vi "Autonomous.vi"() -> ()   [LabVIEW 2020]
doc: "This VI starts when autonomous period begins, and will automatically be terminated when it ends. You can carry out timed or sensor driven operations directly to I/O or to subsystems without needing to return to the caller."
uses:
  <vilib>/Rock Robotics/WPI/Framework/Command Status Info.ctl
  <vilib>/Rock Robotics/WPI/Framework/Completion Status.ctl
  <vilib>/Rock Robotics/WPI/Framework/Completion Notifier.ctl
  Swerve/Implementation/Swerve Operations.ctl
  Swerve/Implementation/Swerve Setpoints.ctl
  <vilib>/Rock Robotics/WPI/Utilities/WPI_GetSetVariantRefNum.vi
  <vilib>/Rock Robotics/Network Tables/NT Read String.vi
panel:
  out "Command Info Out 3":T1
  out "Command Info Out 2":T1
  out "Command Info Out":T1
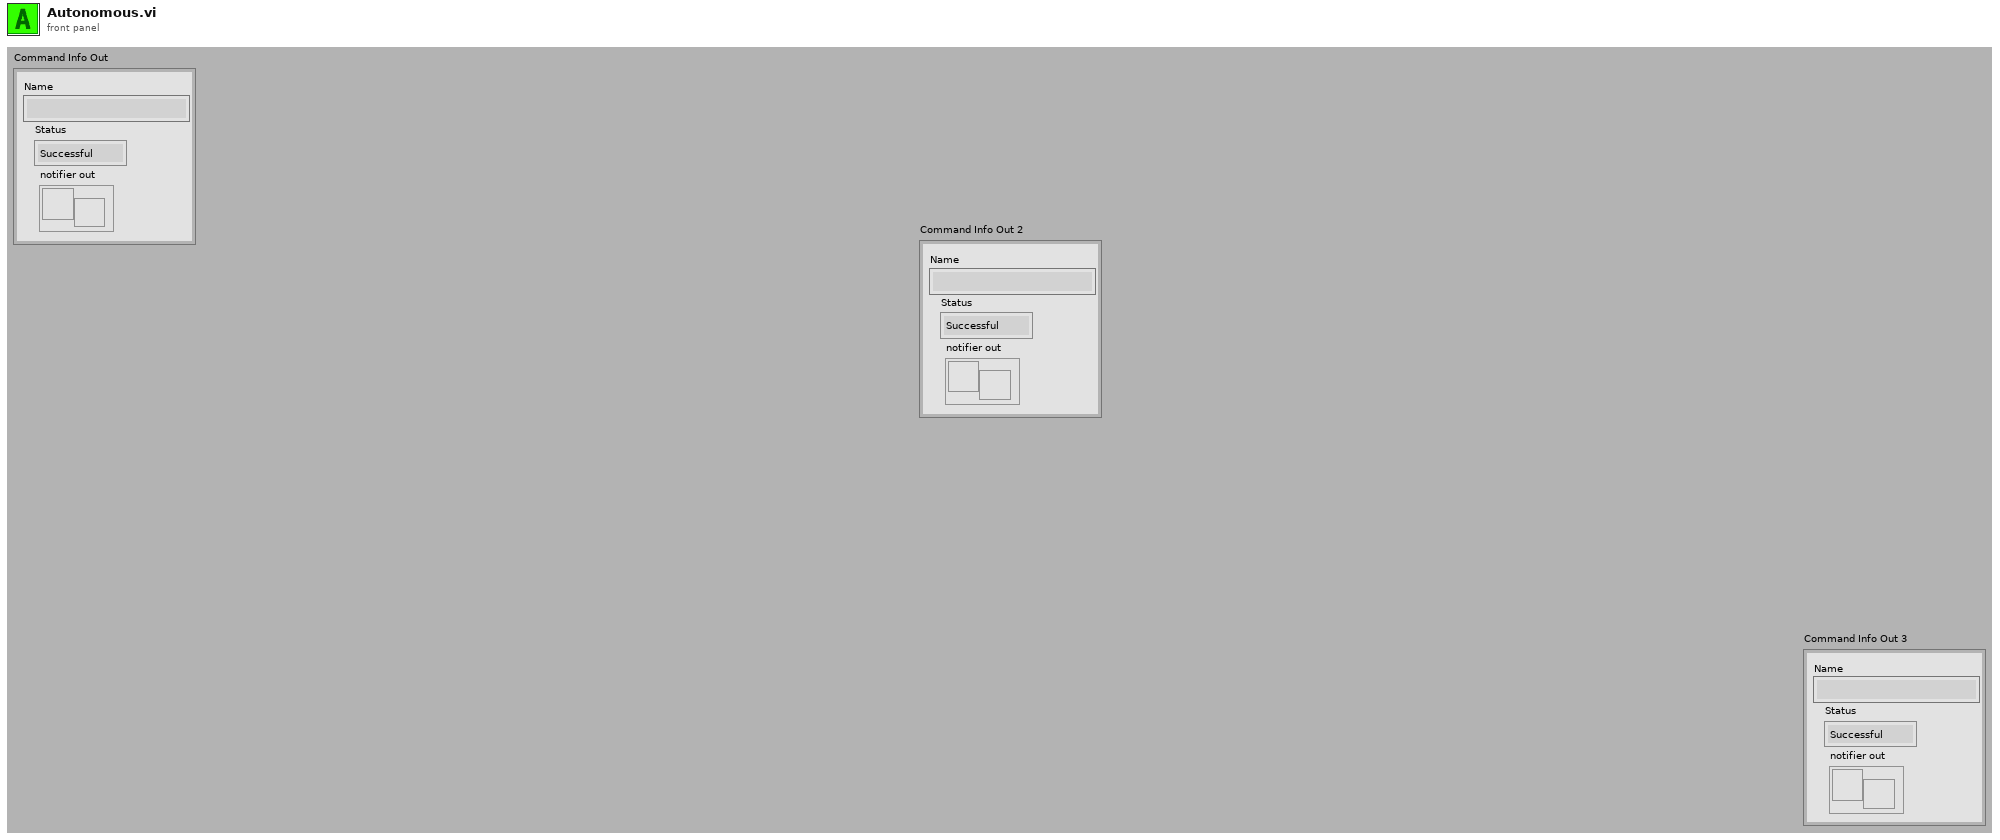
[diagram p1: front panel]
types:
  T1 = typedef "Command Status Info.ctl" = cluster{"Name":string, "Status":T2, "notifier out":T3}
  T2 = typedef "Completion Status.ctl" = enum16{"Successful", "Aborted", "Incomplete"}
  T3 = typedef "Completion Notifier.ctl" = refnum<notifier>
  T4 = typedef "WPI_JoystickDevRef.ctl" = cluster{"Device":T5}
  T5 = typedef "WPI_JoystickDeviceEnum.ctl" = enum16{"USB 0", "USB 1", "USB 2", "USB 3", "USB 4", "USB 5"}
  T6 = typedef "Swerve Setpoints.ctl" = cluster{"Operation":T7, "Gyro":dbl, "X Rotate":dbl, "FWD":dbl, "STR":dbl, "Time":dbl, "Angle":dbl, "Distance":dbl, "Right Trigger":dbl, "Y Rotate":dbl, "Start Angle":dbl}
  T7 = typedef "Swerve Operations.ctl" = enum16{"Reserve", "Read Current", "Immediate", "Direct  Joystick Drive", "Joystick Drive", "Drive for Distance", "Drive for Time", "Turn to Angle", "Drive to Angle(Time)", "Drive to Angle(Distance)"}
  T8 = typedef "WPI_MotorControlDeviceRef.ctl" = cluster{"DeviceStatus":errorcluster, "Type":T9, "PWM":cluster{"PWM Channel":T10, "DeadBand":T11}, "CAN":cluster{"Device Number":u8, "SetOutput VI Ref":variant, "GetOutput VI Ref":variant, "Enable VI Ref":variant, "Disable VI Ref":variant, "Data":variant}, "Invert":bool, "DIO PWM":cluster{"PWM \"Enable\" Channel":T10, "DIOChannel":T12, "PWM Rate":dbl}}
  T9 = typedef "WPI_MotorControlType.ctl" = enum16{"PWM", "CAN", "DIO PWM"}
  T10 = typedef "FPGA_DIOPWMChannel.ctl" = enum8{"PWM 0", "PWM 1", "PWM 2", "PWM 3", "PWM 4", "PWM 5", "PWM 6", "PWM 7", "PWM 8", "PWM 9", "PWM MXP 0", "PWM MXP 1", "PWM MXP 2", "PWM MXP 3", "PWM MXP 4", "PWM MXP 5", "PWM MXP 6", "PWM MXP 7", "PWM MXP 8", "PWM MXP 9", "Invalid"}
  T11 = typedef "WPI_PWMDeadband.ctl" = cluster{"Name":string, "maxPositivePwm":i32, "minPositivePwm":i32, "centerPwm":i32, "maxNegativePwm":i32, "minNegativePwm":i32, "angularRange":u16}
  T12 = typedef "FPGA_DIOChannel.ctl" = enum8{"DIO 0", "DIO 1", "DIO 2", "DIO 3", "DIO 4", "DIO 5", "DIO 6", "DIO 7", "DIO 8", "DIO 9", "DIO MXP 0", "DIO MXP 1", "DIO MXP 2", "DIO MXP 3", "DIO MXP 4", "DIO MXP 5", "DIO MXP 6", "DIO MXP 7", "DIO MXP 8", "DIO MXP 9", "DIO MXP 10", "DIO MXP 11", "DIO MXP 12", "DIO MXP 13", "DIO MXP 14", "DIO MXP 15", "SPI Port CS1", "SPI Port CS2", "SPI Port CS3", "SPI Port MISO", "SPI Port MOSI", "Invalid"}
  T13 = typedef "ADIS16470 Device Reference.ctl" = cluster{"DevStatus":errorcluster, "Hardware Config":T14, "Calibration Complete":refnum<notifier>, "Status Reference":refnum<data-value>, "Data Reference":refnum<data-value>, "Sychronous Process VI":T17, "Cmd FIFO":refnum<k33>, "Source":T18, "Data FIFO":refnum<k33>, "Calibration Time (ms)":u32, "Data Reference":refnum<data-value>}
  T14 = typedef "ADIS16470 Hardware Configuration.ctl" = cluster{"SPI Clock Rate (Hz)":dbl, "IMU SPI Mode (3)":T15, "IMU Reset Pin":T12, "IMU SPI Bus":T16, "IMU Data Ready Pin":T12, "Stall Config":cluster{"Pow2BytesPerRead":u8, "StallTicks":u16, "CsToSclkTicks":u8}}
  T15 = typedef "WPI_SPIMode.ctl" = enum16{"Mode 0 (Clk Idle Low,Sample on Leading)", "Mode 1 (Clk Idle Low,Sample on Trailing)", "Mode 2 (Clk Idle High,Sample on Leading)", "Mode 3 (Clk Idle High,Sample on Trailing)"}
  T16 = typedef "spi_bus.ctl" = enum16{"SPI On-Board, CS0", "SPI On-Board, CS1", "SPI On-Board, CS2", "SPI On-Board, CS3", "SPI MXP", "Invalid"}
  T17 = typedef "ADIS16470 Process.ctl" = refnum<vi>
  T18 = typedef "FPGA_CounterEncoderSourceConvertionLVSourceType.ctl" = cluster{"DevStatus":errorcluster, "AnalogTriggerMode?":bool, "DigitalMode":cluster{"DIO Channel":T19}, "AnalogTriggerMode":cluster{"AnalogTriggerIndex":T20, "OutputType":T21}}
  T19 = typedef "FPGA_DIODigitalSourceChannel.ctl" = enum8{"DIO 0", "DIO 1", "DIO 2", "DIO 3", "DIO 4", "DIO 5", "DIO 6", "DIO 7", "DIO 8", "DIO 9", "DIO MXP 0", "DIO MXP 1", "DIO MXP 2", "DIO MXP 3", "DIO MXP 4", "DIO MXP 5", "DIO MXP 6", "DIO MXP 7", "DIO MXP 8", "DIO MXP 9", "DIO MXP 10", "DIO MXP 11", "DIO MXP 12", "DIO MXP 13", "DIO MXP 14", "DIO MXP 15", "SPI Port CS1", "SPI Port CS2", "SPI Port CS3", "SPI Port MISO", "SPI Port MOSI", "Disabled"}
  T20 = typedef "FPGA_AnalogTriggerIndex.ctl" = enum8{"Trig 0", "Trig 1", "Trig 2", "Trig 3", "Trig 4", "Trig 5", "Trig 6", "Trig 7", "Invalid"}
  T21 = typedef "FPGA_AnalogTriggerOutType.ctl" = enum16{"InWindow", "TriggerState", "Rising", "Falling"}
  T22 = typedef "ADIS16470 Data.ctl" = cluster{"XAngle":dbl, "YAngle":dbl, "ZAngle":dbl}
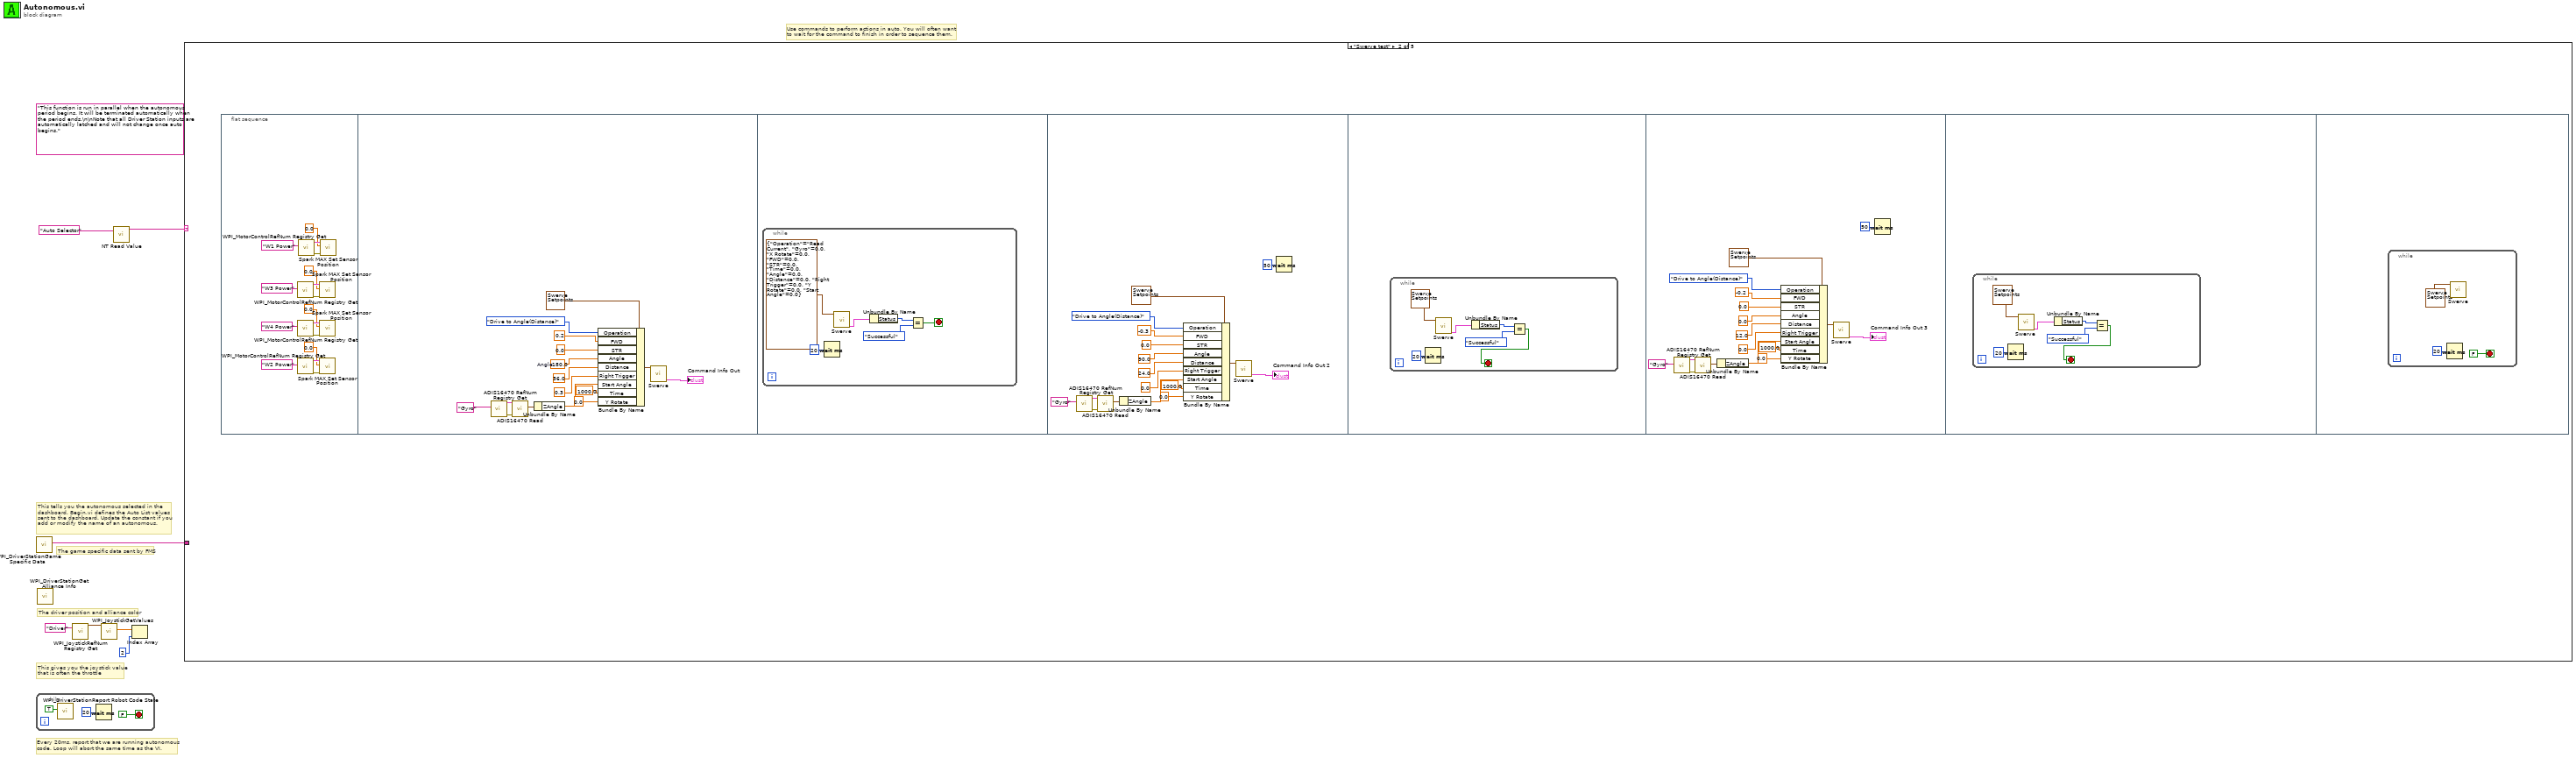
[diagram p0: block diagram]
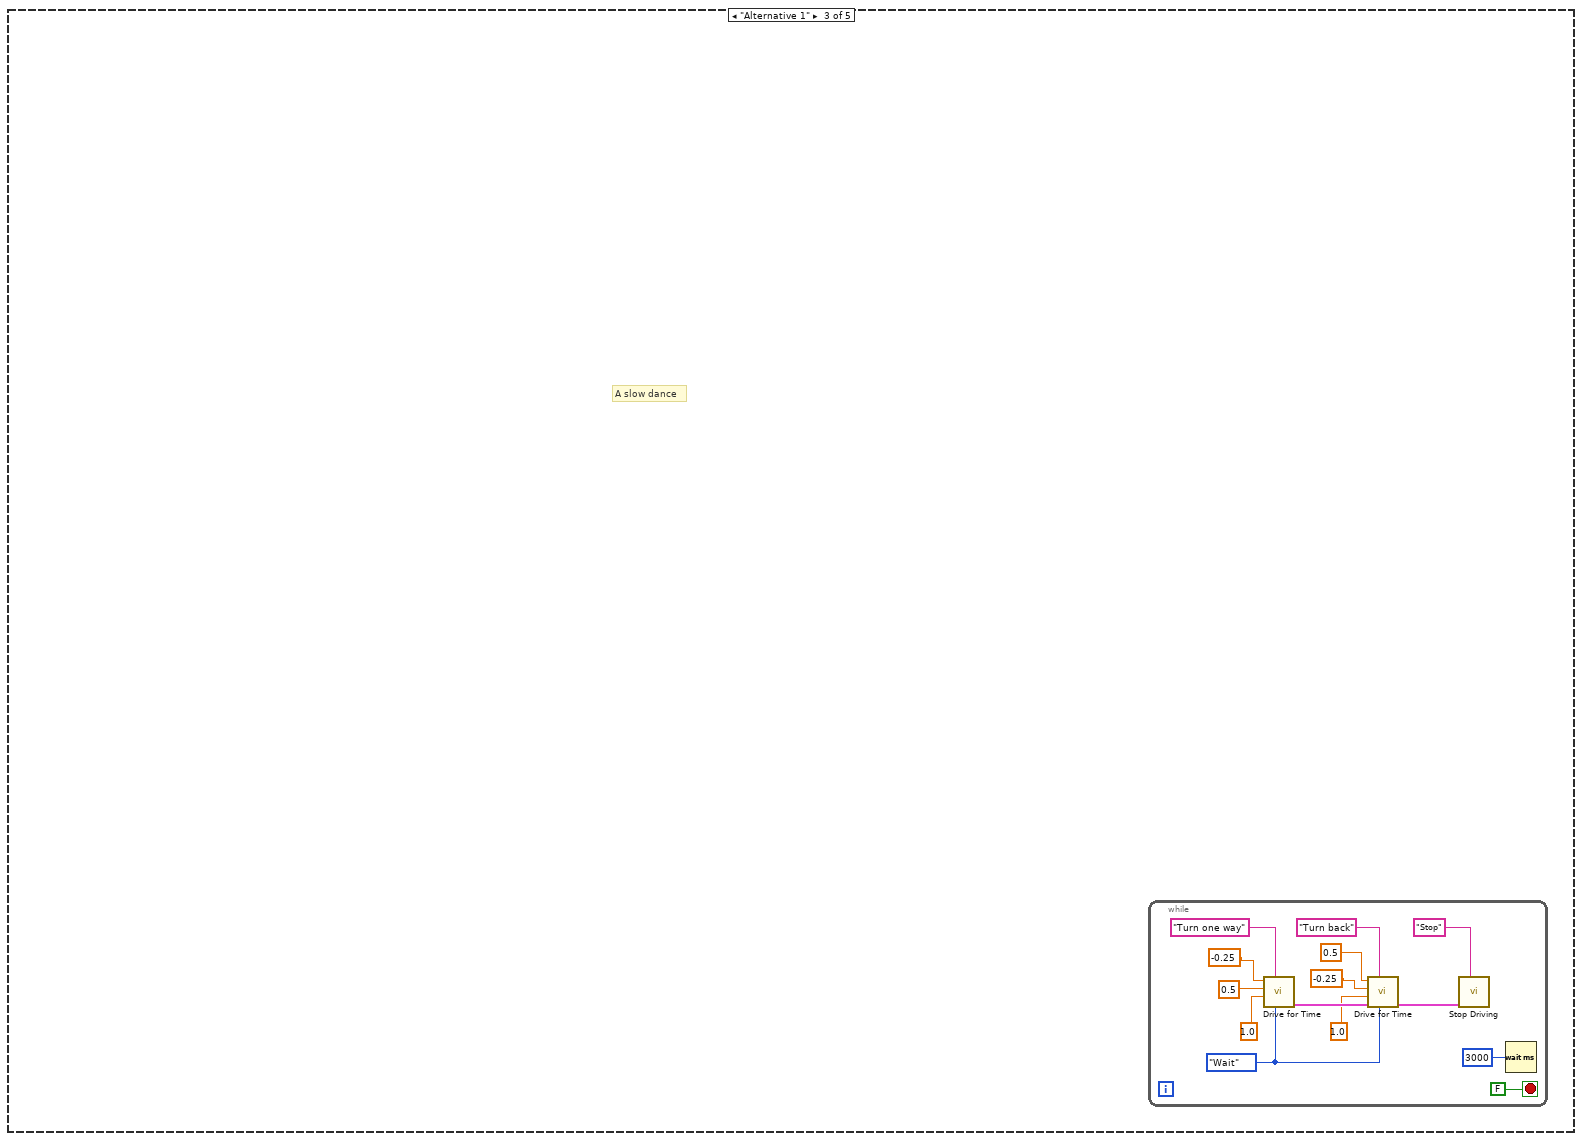
[diagram p3: hidden frame]
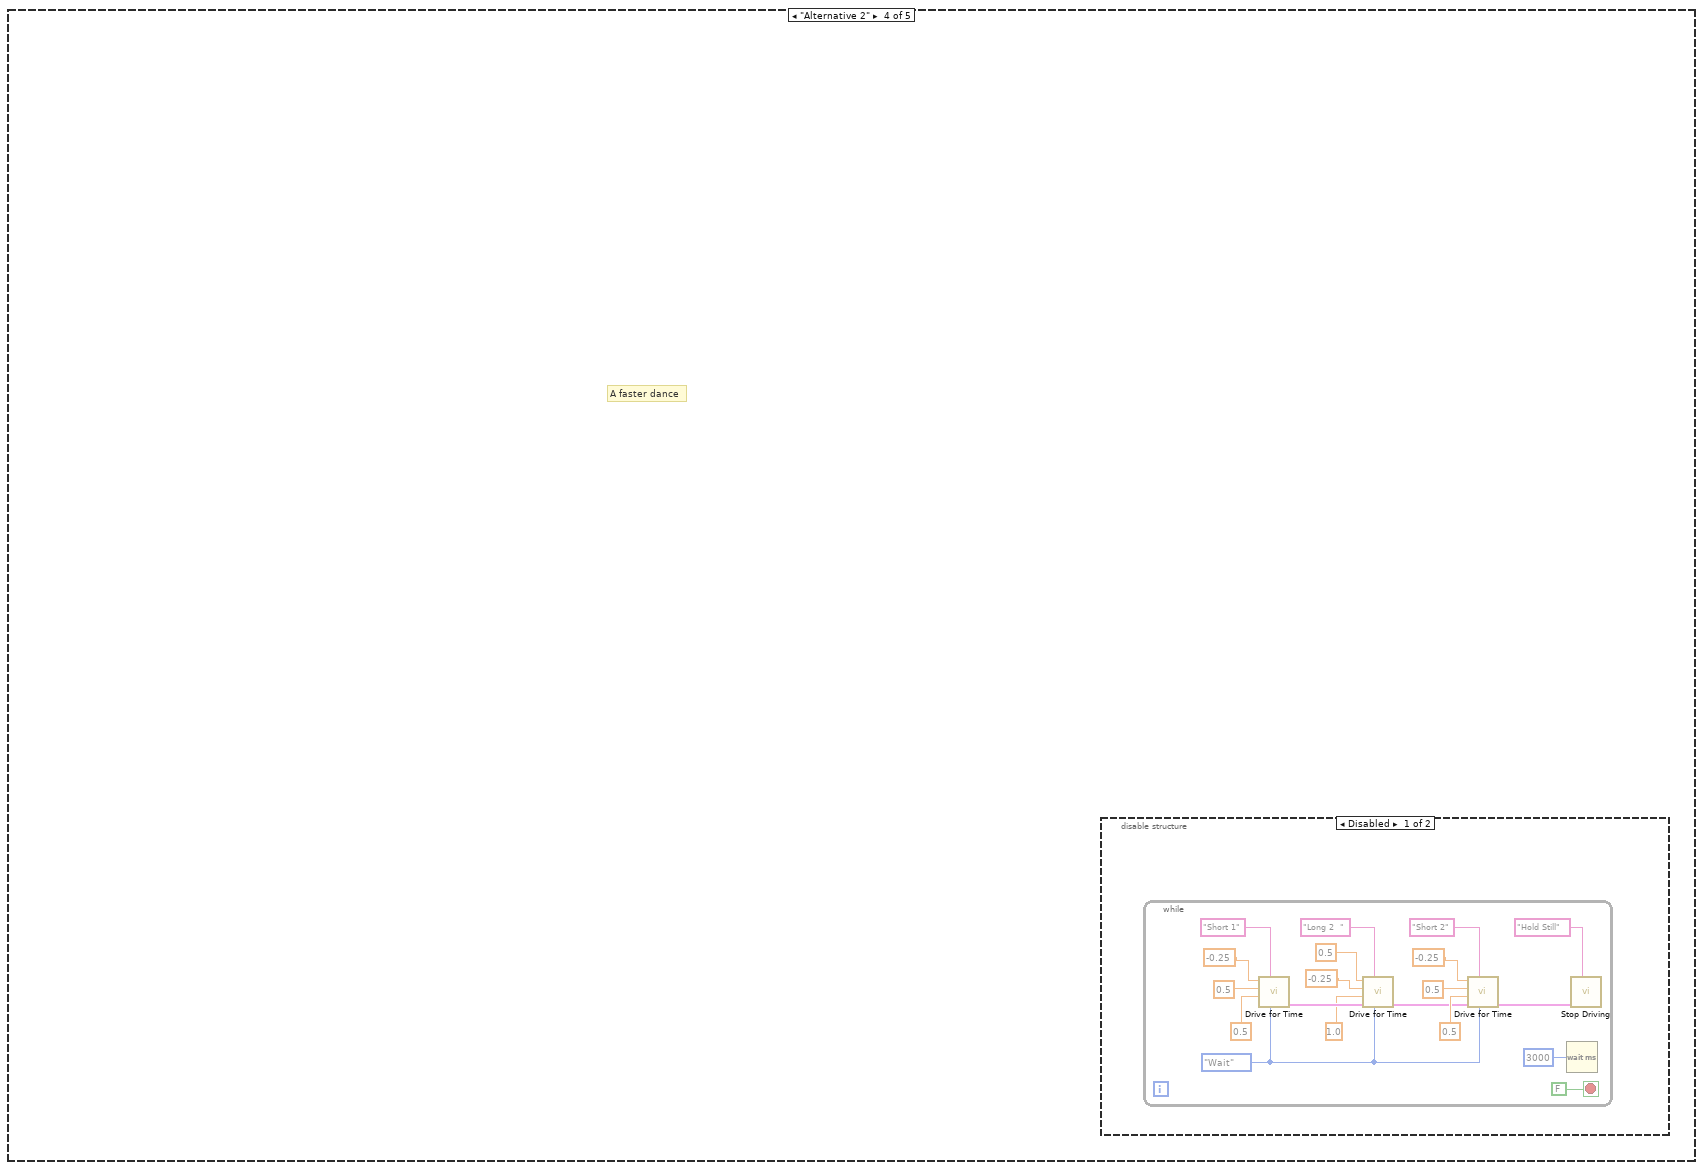
[diagram p4: hidden frame]
diagram:
  (unwired) "This function is run in parallel when the autonomous period begins. It will be terminated automatically when the period ends.\n\nNote that all Driver Station inputs are automatically latched and will not change once auto begins."
  # "The game specific data sent by FMS"
  # "This tells you the autonomous selected in the \ndashboard. Begin.vi defines the Auto List values\nsent to the dashboard. Update the constant if you\nadd or modify the name of an autonomous."
  # "Every 20ms, report that we are running autonomous\ncode. Loop will abort the same time as the VI."
  # "This gives you the joystick value\nthat is often the throttle"
  # "Use commands to perform actions in auto. You will often want\nto wait for the command to finish in order to sequence them."
  # "The driver position and alliance color"
  n1 = call <vilib>:"WPI_DriverStationGame Specific Data.vi"() -> ("Game Specific Data"=w1:string)  [unwired: 11 in]
  n2 = while {
    stop <- FALSE stop-if-true
    n3 = call <vilib>:"WPI_DriverStationReport Robot Code State.vi"("Autonomous"=TRUE) -> ()  [unwired: 10 in, 1 out]
    n4 = Wait (ms)(milliseconds to wait=u32 20) -> ()  [unwired: 1 out]
  }
  n5 = call <vilib>:"WPI_DriverStationGet Alliance Info.vi"() -> ()  [unwired: 12 out]
  n6 = call <vilib>:"WPI_JoystickRefNum Registry Get.vi"("refnum name"="Driver") -> ("JoystickDevRef"=w6:T4)  [unwired: 1 in, 9 out]
  n7 = call <vilib>:"WPI_JoystickGetValues.vi"("JoystickDevRef"=w6) -> ("Axes"=w5:dbl[])  [unwired: 6 in, 4 out]
  n8 = call-poly <vilib>:"NT Read Value.vi"("Name"="Auto Selector") -> ("String"=w2:string)  [unwired: 9 in, 1 out]
  n9 = Index Array(array=w5, index=2) -> ()  [unwired: 1 out]
  n10 = case shown="\"Swerve test\"" w2 {
    tunnel: w1 -> [_ _ _ _ _]
    frame Default {
      # "You can put your main auto here, or you can right-click on the case and make any\nother frame be the default case."
      # "This is the frame that will execute if no selection is made, or if it is not recognized"
    }
    frame "Swerve test" {
      n11 = flat-sequence {
        frame #0 {
          n12 = call <vilib>:"WPI_MotorControlRefNum Registry Get.vi"("refnum name"="W3 Power") -> ("error out"=w23:errorcluster, "MotorControlDevRef"=w24:T8)  [unwired: 9 in]
          n13 = call <vilib>:"WPI_MotorControlRefNum Registry Get.vi"("refnum name"="W4 Power") -> ("error out"=w25:errorcluster, "MotorControlDevRef"=w26:T8)  [unwired: 9 in]
          n14 = call <vilib>:"WPI_MotorControlRefNum Registry Get.vi"("refnum name"="W2 Power") -> ("error out"=w21:errorcluster, "MotorControlDevRef"=w22:T8)  [unwired: 9 in]
          n15 = call <vilib>:"WPI_MotorControlRefNum Registry Get.vi"("refnum name"="W1 Power") -> ("error out"=w19:errorcluster, "MotorControlDevRef"=w20:T8)  [unwired: 9 in]
          n16 = call <vilib>:"Spark MAX Set Sensor Position.vi"("error in"=w23, "Position"=0.0, "MotorControlDeviceRef"=w24) -> ()  [unwired: 7 in, 2 out]
          n17 = call <vilib>:"Spark MAX Set Sensor Position.vi"("error in"=w25, "Position"=0.0, "MotorControlDeviceRef"=w26) -> ()  [unwired: 7 in, 2 out]
          n18 = call <vilib>:"Spark MAX Set Sensor Position.vi"("error in"=w21, "Position"=0.0, "MotorControlDeviceRef"=w22) -> ()  [unwired: 7 in, 2 out]
          n19 = call <vilib>:"Spark MAX Set Sensor Position.vi"("error in"=w19, "Position"=0.0, "MotorControlDeviceRef"=w20) -> ()  [unwired: 7 in, 2 out]
        }
        frame #1 {
          w33 = 180.0  # Angle
          n20 = call <vilib>:"ADIS16470 RefNum Registry Get.vi"("refnum name"="Gyro") -> ("error out"=w39:errorcluster, "ADIS16470DevRef out"=w38:T13)  [unwired: 9 in]
          n21 = call <vilib>:"ADIS16470 Read.vi"("error in (no error)"=w39, "ADIS16470DevRef"=w38) -> ("ADIS16470 Value"=w37:T22)  [unwired: 6 in, 3 out]
          n22 = Unbundle By Name(w37) -> ("ZAngle"=w35:dbl)
          n23 = Bundle By Name(cluster=T6 {"Operation"=enum."Reserve", "Gyro"=0.0, "X Rotate"=0.0, "FWD"=0.0, "STR"=0.0, "Time"=0.0, "Angle"=0.0, "Distance"=0.0, "Right Trigger"=0.0, "Y Rotate"=0.0, "Start Angle"=0.0} ("SubSystem Data"), "Operation"=Swerve_Operations."Drive to Angle(Distance)", "FWD"=0.2, "STR"=0.0, "Angle"=w33, "Distance"=36.0, "Right Trigger"=0.3, "Start Angle"=w35, "Time"=1000.0, "Y Rotate"=0.0) -> (w42:T6)
          n24 = call "Swerve.vi"("SubSystem Data"=w42) -> ("Command Info Out"=→"Command Info Out":T1)  [unwired: 10 in]
        }
        frame #2 {
          n25 = while {
            stop <- w43 stop-if-true
            n26 = Wait (ms)(milliseconds to wait=u32 20) -> ()  [unwired: 1 out]
            n27 = call "Swerve.vi"("SubSystem Data"=T6 {"Operation"=enum."Read Current", "Gyro"=0.0, "X Rotate"=0.0, "FWD"=0.0, "STR"=0.0, "Time"=0.0, "Angle"=0.0, "Distance"=0.0, "Right Trigger"=0.0, "Y Rotate"=0.0, "Start Angle"=0.0}) -> ("Command Info Out"=w46:T1)  [unwired: 10 in]
            n28 = Unbundle By Name(w46) -> ("Status"=w44:T2)
            n29 = Equal?(x=w44, y=Completion_Status."Successful") -> (x = y?=w43:bool)
          }
        }
        frame #3 {
          n30 = call <vilib>:"ADIS16470 RefNum Registry Get.vi"("refnum name"="Gyro") -> ("error out"=w62:errorcluster, "ADIS16470DevRef out"=w61:T13)  [unwired: 9 in]
          n31 = call <vilib>:"ADIS16470 Read.vi"("error in (no error)"=w62, "ADIS16470DevRef"=w61) -> ("ADIS16470 Value"=w60:T22)  [unwired: 6 in, 3 out]
          n32 = Unbundle By Name(w60) -> ("ZAngle"=w58:dbl)
          n33 = Bundle By Name(cluster=T6 {"Operation"=enum."Reserve", "Gyro"=0.0, "X Rotate"=0.0, "FWD"=0.0, "STR"=0.0, "Time"=0.0, "Angle"=0.0, "Distance"=0.0, "Right Trigger"=0.0, "Y Rotate"=0.0, "Start Angle"=0.0} ("SubSystem Data"), "Operation"=Swerve_Operations."Drive to Angle(Distance)", "FWD"=-0.3, "STR"=0.0, "Angle"=90.0, "Distance"=24.0, "Right Trigger"=0.0, "Start Angle"=w58, "Time"=1000.0, "Y Rotate"=0.0) -> (w65:T6)
          n34 = call "Swerve.vi"("SubSystem Data"=w65) -> ("Command Info Out"=→"Command Info Out 2":T1)  [unwired: 10 in]
          n35 = Wait (ms)(milliseconds to wait=u32 50) -> ()  [unwired: 1 out]
        }
        frame #4 {
          n36 = while {
            stop <- w66 stop-if-true
            n37 = Wait (ms)(milliseconds to wait=u32 20) -> ()  [unwired: 1 out]
            n38 = call "Swerve.vi"("SubSystem Data"=T6 {"Operation"=enum."Read Current", "Gyro"=0.0, "X Rotate"=0.0, "FWD"=0.0, "STR"=0.0, "Time"=0.0, "Angle"=0.0, "Distance"=0.0, "Right Trigger"=0.0, "Y Rotate"=0.0, "Start Angle"=0.0}) -> ("Command Info Out"=w69:T1)  [unwired: 10 in]
            n39 = Unbundle By Name(w69) -> ("Status"=w67:T2)
            n40 = Equal?(x=w67, y=Completion_Status."Successful") -> (x = y?=w66:bool)
          }
        }
        frame #5 {
          n41 = call <vilib>:"ADIS16470 RefNum Registry Get.vi"("refnum name"="Gyro") -> ("error out"=w85:errorcluster, "ADIS16470DevRef out"=w84:T13)  [unwired: 9 in]
          n42 = call <vilib>:"ADIS16470 Read.vi"("error in (no error)"=w85, "ADIS16470DevRef"=w84) -> ("ADIS16470 Value"=w83:T22)  [unwired: 6 in, 3 out]
          n43 = Unbundle By Name(w83) -> ("ZAngle"=w81:dbl)
          n44 = Bundle By Name(cluster=T6 {"Operation"=enum."Reserve", "Gyro"=0.0, "X Rotate"=0.0, "FWD"=0.0, "STR"=0.0, "Time"=0.0, "Angle"=0.0, "Distance"=0.0, "Right Trigger"=0.0, "Y Rotate"=0.0, "Start Angle"=0.0} ("SubSystem Data"), "Operation"=Swerve_Operations."Drive to Angle(Distance)", "FWD"=-0.2, "STR"=0.0, "Angle"=0.0, "Distance"=12.0, "Right Trigger"=0.0, "Start Angle"=w81, "Time"=1000.0, "Y Rotate"=0.0) -> (w88:T6)
          n45 = call "Swerve.vi"("SubSystem Data"=w88) -> ("Command Info Out"=→"Command Info Out 3":T1)  [unwired: 10 in]
          n46 = Wait (ms)(milliseconds to wait=u32 50) -> ()  [unwired: 1 out]
        }
        frame #6 {
          n47 = while {
            stop <- w89 stop-if-true
            n48 = Wait (ms)(milliseconds to wait=u32 20) -> ()  [unwired: 1 out]
            n49 = call "Swerve.vi"("SubSystem Data"=T6 {"Operation"=enum."Read Current", "Gyro"=0.0, "X Rotate"=0.0, "FWD"=0.0, "STR"=0.0, "Time"=0.0, "Angle"=0.0, "Distance"=0.0, "Right Trigger"=0.0, "Y Rotate"=0.0, "Start Angle"=0.0}) -> ("Command Info Out"=w92:T1)  [unwired: 10 in]
            n50 = Unbundle By Name(w92) -> ("Status"=w90:T2)
            n51 = Equal?(x=w90, y=Completion_Status."Successful") -> (x = y?=w89:bool)
          }
        }
        frame #7 {
          n52 = while {
            stop <- FALSE stop-if-true
            n53 = Wait (ms)(milliseconds to wait=u32 20) -> ()  [unwired: 1 out]
            n54 = call "Swerve.vi"("SubSystem Data"=T6 {"Operation"=enum."Joystick Drive", "Gyro"=0.0, "X Rotate"=0.0, "FWD"=0.0, "STR"=0.0, "Time"=0.0, "Angle"=0.0, "Distance"=0.0, "Right Trigger"=0.0, "Y Rotate"=0.0, "Start Angle"=0.0}) -> ()  [unwired: 10 in, 1 out]
          }
        }
      }
    }
    frame "Alternative 1" {
      # "A slow dance"
      n55 = while {
        stop <- FALSE stop-if-true
        w102 = enum16{"Start", "Wait"}."Wait" ("Synchronication")
        n56 = call "Drive for Time.vi"("Synchronization"=w102, "Description"="Turn one way", "Seconds"=1.0 ("Delay (s)"), "Right Speed"=0.5 ("X axis value"), "Left Speed"=-0.25 ("X axis value")) -> ("Command Info Out"=w111:T1)  [unwired: 6 in]
        n57 = call "Drive for Time.vi"("Synchronization"=w102, "Description"="Turn back", "Command Info In"=w111, "Seconds"=1.0 ("Delay (s)"), "Right Speed"=-0.25 ("X axis value"), "Left Speed"=0.5 ("X axis value")) -> ("Command Info Out"=w101:T1)  [unwired: 5 in]
        n58 = call "Stop Driving.vi"("Description"="Stop", "Command Info In"=w101) -> ()  [unwired: 9 in, 1 out]
        n59 = Wait (ms)(milliseconds to wait=u32 3000 ("millisecond timer value")) -> ()  [unwired: 1 out]
      }
    }
    frame "Alternative 2" {
      # "A faster dance"
      n60 = disable-structure shown="Disabled" {
        frame Disabled {
          n61 = while {
            stop <- FALSE stop-if-true
            w112 = enum16{"Start", "Wait"}."Wait" ("Synchronication")
            n62 = call "Drive for Time.vi"("Synchronization"=w112, "Description"="Short 1", "Seconds"=0.5 ("Delay (s)"), "Right Speed"=0.5 ("X axis value"), "Left Speed"=-0.25 ("X axis value")) -> ("Command Info Out"=w130:T1)  [unwired: 6 in]
            n63 = call "Drive for Time.vi"("Synchronization"=w112, "Description"="Long 2  ", "Command Info In"=w130, "Seconds"=1.0 ("Delay (s)"), "Right Speed"=-0.25 ("X axis value"), "Left Speed"=0.5 ("X axis value")) -> ("Command Info Out"=w114:T1)  [unwired: 5 in]
            n64 = call "Drive for Time.vi"("Synchronization"=w112, "Description"="Short 2", "Command Info In"=w114, "Seconds"=0.5 ("Delay (s)"), "Right Speed"=0.5 ("X axis value"), "Left Speed"=-0.25 ("X axis value")) -> ("Command Info Out"=w113:T1)  [unwired: 5 in]
            n65 = Wait (ms)(milliseconds to wait=u32 3000 ("millisecond timer value")) -> ()  [unwired: 1 out]
            n66 = call "Stop Driving.vi"("Description"="Hold Still", "Command Info In"=w113) -> ()  [unwired: 9 in, 1 out]
          }
        }
        frame Enabled {
        }
      }
    }
    frame "Your Turn" {
    }
  }
